vi "c REV Lib Error From Code.vi"(8 "error in (no error)":errorcluster, 11 "code":u32(ring) items=["c_REVLibError_None", "c_REVLibError_General", "c_REVLibError_CANTimeout", "c_REVLibError_NotImplemented", "c_REVLibError_HAL", "c_REVLibError_CantFindFirmware", "c_REVLibError_FirmwareTooOld", "c_REVLibError_FirmwareTooNew", "c_REVLibError_ParamInvalidID", "c_REVLibError_ParamMismatchType", "c_REVLibError_ParamAccessMode", "c_REVLibError_ParamInvalid", "c_REVLibError_ParamNotImplementedDeprecated", "c_REVLibError_FollowConfigMismatch", "c_REVLibError_Invalid", "c_REVLibError_SetpointOutOfRange", "c_REVLibError_Unknown", "c_REVLibError_CANDisconnected", "c_REVLibError_DuplicateCANId", "c_REVLibError_InvalidCANId", "c_REVLibError_SparkMaxDataPortAlreadyConfiguredDifferently", "c_REVLibError_SparkFlexBrushedWithoutDock", "c_REVLibError_NumCodes"]) -> (0 "error out":errorcluster, 3 "function return":string)   [LabVIEW 2023, in "REVLibDriver.lvlib"]
doc: "const char* c_REVLib_ErrorFromCode(c_REVLib_ErrorCode code);"
uses:
  REVLibDriver.lvlib
  REVLibDriver.dll
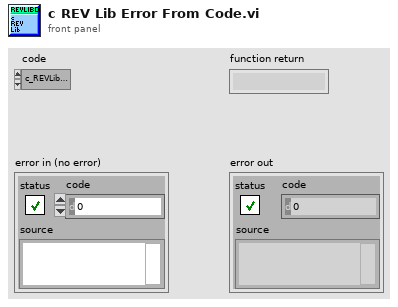
[diagram p1: front panel]
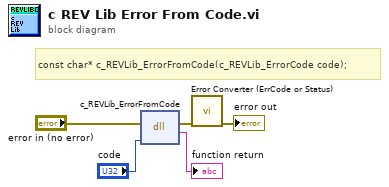
[diagram p0: block diagram]
diagram:
  # "const char* c_REVLib_ErrorFromCode(c_REVLib_ErrorCode code);"
  n1 = dll-call lib="REVLibDriver.*" fn="c_REVLib_ErrorFromCode"(error in="error in (no error)", "code"="code") -> (error out=w2:errorcluster, →"function return":string)  [unwired: 3 in, 1 out]
  n2 = call "Error Converter (ErrCode or Status).vi"("error in (no error)"=w2) -> ("error out"=→"error out":errorcluster)  [unwired: 10 in]
